vi "Draw_Point.vi"(6 "color":u32(colorbox)=65316, 8 "Draw?":bool=TRUE, 9 "point":cluster{"x":dbl, "y":dbl}, 11 "picture in":picture) -> (3 "new picture":picture)   [LabVIEW 2022 SP3]
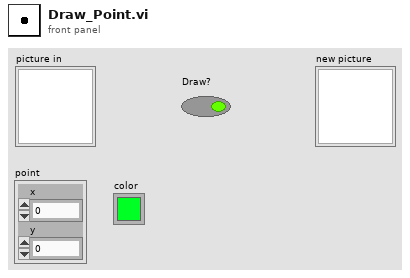
[diagram p1: front panel]
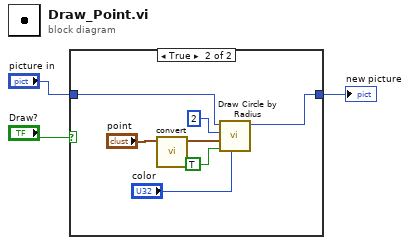
[diagram p0: block diagram]
diagram:
  n1 = case shown="True" "Draw?" {
    tunnel: "picture in" -> [w4 w9]
    tunnel: [w4 w8] -> w2
    frame False {
    }
    frame True {
      n2 = call "convert.vi"("point"="point") -> ("scaled"=w11:cluster{"x":dbl, "y":dbl})  [unwired: 10 in]
      n3 = call <vilib>:"Draw Circle by Radius.vi"("color(black)"="color", "fill?(F)"=TRUE, "pixel center"=w11, "radius"=i16 2, "picture"=w9) -> ("new picture"=w8:picture)  [unwired: 6 in]
    }
  }
  "new picture" <- w2
